vi "Fetch DB List.vi"(8 "error in (no error)":errorcluster, 9 "Data Type":string[][](array[string]), 10 "SQL Query":string, 11 "Refnum in":T1) -> (0 "error out":errorcluster, 2 "Data Result":string[](array[combo]), 3 "Refnum out":T1)   [LabVIEW 2026, in "Database.lvlib"]
uses:
  Database.lvlib
  <vilib>/addons/database/Connection.llb/Conn ObjectReference.ctl
  <vilib>/addons/database/Connection.llb/Conn Execute.vi
  <vilib>/addons/database/Recordset.llb/Rec Fetch Recordset Data (R).vi
  <vilib>/addons/database/Recordset.llb/Rec Destroy - Connection.vi
  <vilib>/addons/database/NI_Database_API.lvlib
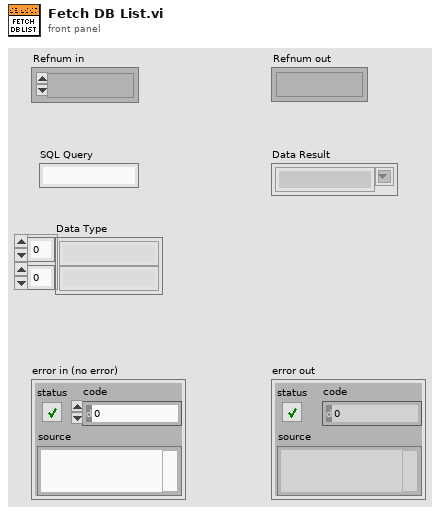
[diagram p1: front panel]
types:
  T1 = typedef "NI_Database_API.lvlib/Conn ObjectReference.ctl" = refnum<k1>
  T2 = typedef "NI_Database_API.lvlib/Rec ObjectReference.ctl" = refnum<k1>
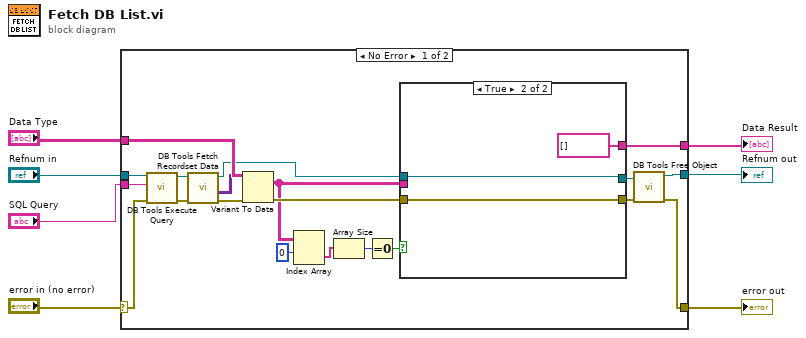
[diagram p0: block diagram]
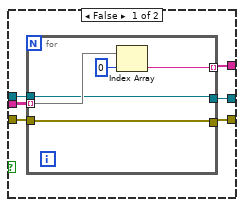
[diagram p2: hidden frame]
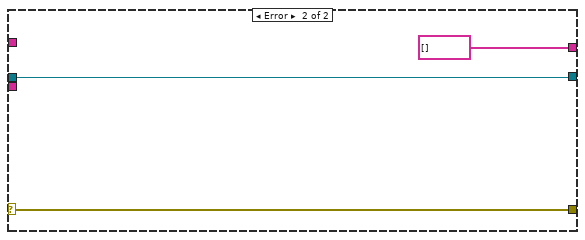
[diagram p3: hidden frame]
diagram:
  n1 = case shown="No Error" "error in (no error)" {
    selector: "error in (no error)" -> [w13 w44]
    tunnel: [w27 string[] []] -> w7
    tunnel: [w26 w43] -> w6
    tunnel: "Data Type" -> [w22 _]
    tunnel: "SQL Query" -> [w16 _]
    tunnel: [w15 w44] -> w3
    tunnel: "Refnum in" -> [w14 w43]
    frame No Error {
      n2 = call-poly <vilib>:"DB Tools Execute Query.vi"("error in (no error)"=w13, "SQL query"=w16, "connection reference"=w14) -> ("error out"=w17:errorcluster, "recordset reference"=w18:T2)  [unwired: 5 in]
      n3 = call-poly <vilib>:"DB Tools Fetch Recordset Data.vi"("error in (no error)"=w17, "recordset reference"=w18) -> ("error out"=w19:errorcluster, "recordset data"=w20:variant[][], "recordset reference out"=w21:T2)  [unwired: 3 in]
      n4 = Variant To Data(error in=w19, type=w22, Variant=w20) -> (data=w12:string[][], error out=w23:errorcluster)
      n5 = Index Array(array=w12, index (row)=0) -> (element=w10:string[])  [unwired: 1 in]
      n6 = Array Size(array=w10) -> (size(s)=w9:i32)
      n7 = Equal To 0?(x=w9) -> (x = 0?=w8:bool)
      n8 = case shown="True" w8 {
        tunnel: [w33 string[] []] -> w27
        tunnel: w12 -> [w32 _]
        tunnel: [w31 w40] -> w25
        tunnel: [w30 w41] -> w24
        tunnel: w23 -> [w29 w40]
        tunnel: w21 -> [w28 w41]
        frame False {
          n9 = for {
            tunnel: w29 -> [w35]
            tunnel: w28 -> [w34]
            tunnel: w32 -> [w37] mode=indexing
            tunnel: [w36] -> w33 mode=indexing
            tunnel: [w34] -> w30
            tunnel: [w35] -> w31
            n10 = Index Array(array=w37, index=0) -> (element=w36:string)
          }
        }
        frame True {
        }
      }
      n11 = call-poly <vilib>:"DB Tools Free Object.vi"("error in (no error)"=w25, "recordset reference"=w24) -> ("error out"=w15:errorcluster, "connection reference"=w26:T1)  [unwired: 8 in]
    }
    frame Error {
    }
  }
  "Data Result" <- w7
  "Refnum out" <- w6
  "error out" <- w3
